vi "RichToFlatnixnet_grpc_EnetFrameResponse.vi"(5 "OutputClusterType":T1, 11 "InputCluster":T4) -> (3 "OutputCluster":T1)   [LabVIEW 2025, in "xnet-grpc_client.lvlib"]
uses:
  nixnet_grpc_EnetFrameResponse.ctl
  nixnet_grpc_EnetFrameType.ctl
  nixnet_grpc_EnetFlags.ctl
  nixnet_grpc_EnetFrameResponse_Flat.ctl
  xnet-grpc_client.lvlib
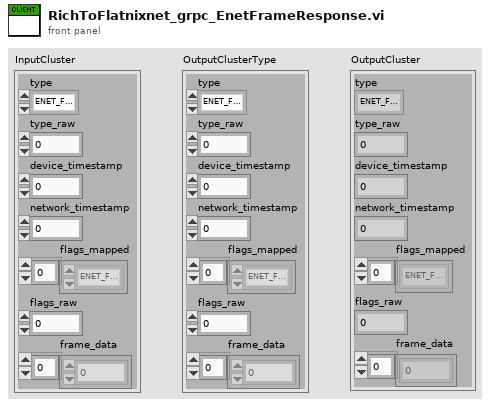
[diagram p1: front panel]
types:
  T1 = typedef "xnet-grpc_client.lvlib/nixnet_grpc_EnetFrameResponse_Flat.ctl" = cluster{"type":T2, "type_raw":u32, "device_timestamp":u64, "network_timestamp":u64, "flags_mapped":T3[], "flags_raw":u32, "frame_data":u8[]}
  T2 = typedef "xnet-grpc_client.lvlib/nixnet_grpc_EnetFrameType.ctl" = enum32{"ENET_FRAME_TYPE_DATA", "ENET_FRAME_TYPE_DELAY", "ENET_FRAME_TYPE_FUTURE_TIME_WAIT"}
  T3 = typedef "xnet-grpc_client.lvlib/nixnet_grpc_EnetFlags.ctl" = enum32{"ENET_FLAGS_UNSPECIFIED", "ENET_FLAGS_TRANSMIT", "ENET_FLAGS_RECEIVE", "ENET_FLAGS_NETWORK_SYNCED", "ENET_FLAGS_ERROR"}
  T4 = typedef "xnet-grpc_client.lvlib/nixnet_grpc_EnetFrameResponse.ctl" = cluster{"type":T2, "type_raw":u32, "device_timestamp":u64, "network_timestamp":u64, "flags_mapped":T3[], "flags_raw":u32, "frame_data":u8[]}
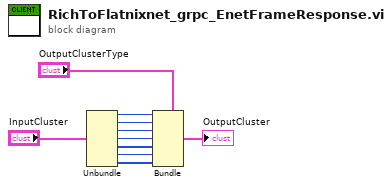
[diagram p0: block diagram]
diagram:
  n1 = Unbundle "Unbundle"("InputCluster") -> ("type"=w7:T2, "type_raw"=w6:u32, "device_timestamp"=w5:u64, "network_timestamp"=w4:u64, "flags_mapped"=w3:T3[], "flags_raw"=w2:u32, "frame_data"=w1:u8[])
  n2 = Bundle "Bundle"(cluster="OutputClusterType", "type"=w7, "type_raw"=w6, "device_timestamp"=w5, "network_timestamp"=w4, "flags_mapped"=w3, "flags_raw"=w2, "frame_data"=w1) -> (→"OutputCluster":T1)
